vi "NF87xx.evt call STOP.vi"(0 "i ref in":refnum<vi>, 1 "Instance":string="N/A", 2 "System (N/A)":string="N/A", 5 "error in (no error)":errorcluster) -> (14 "i ref out":refnum<vi>, 19 "error out":errorcluster)   [LabVIEW 2014, in "NF87XX.lvlib"]
doc: "This VI sets the \"Stop\" case by a simple call. If \"System (N/A)\" is not connected (or \"N/A\" chosen), it acts on all systems connected to the instance, otherwise on the system only."
uses:
  NF87XX.lvlib
  CSCore/CSSystem/CoreLib/CoreLib.string 2 byte array.vi
  CSCore/BaseProcess/BaseProcess.lvlib
  CSCore/CSSystem/CoreLib/CoreLib.lvlib
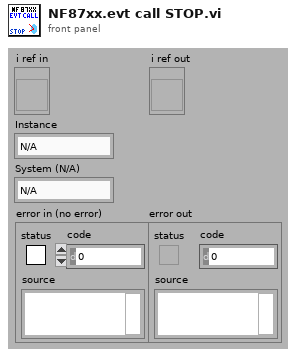
[diagram p1: front panel]
types:
  T1 = enum16{"simple", "synchronous", "asynchronous", "notification"}
  T2 = typedef "CoreDefs.rawDataType.ctl" = i8[]
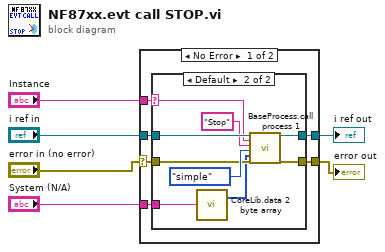
[diagram p0: block diagram]
diagram:
  n1 = case shown="No Error" "error in (no error)" {
    selector: "error in (no error)" -> [w8 w24]
    tunnel: [w12 w25] -> w6
    tunnel: [w11 w24] -> w5
    tunnel: "i ref in" -> [w10 w25]
    tunnel: "Instance" -> [w9 _]
    tunnel: "System (N/A)" -> [w7 _]
    frame No Error {
      n2 = case shown="Default" w9 {
        selector: w9 -> [_ w20]
        tunnel: [w14 w23] -> w12
        tunnel: [w13 w22] -> w11
        tunnel: w10 -> [w14 w21]
        tunnel: w8 -> [w13 w16]
        tunnel: w7 -> [_ w17]
        frame "N/A" {
        }
        frame Default {
          n3 = call-poly "CoreLib.data 2 byte array.vi"("string"=w17) -> ("byteArray out"=w15:T2)  [unwired: 18 in]
          n4 = call "BaseProcess.call process 1.vi"("i ref in"=w21, "Object"=w20, "Selector"="Stop", "CallType"=T1."simple", "Data"=w15, "error in (no error)"=w16) -> ("i ref out"=w23:refnum<vi>, "error out"=w22:errorcluster)  [unwired: 11 in, 1 out]
        }
      }
    }
    frame Error {
    }
  }
  "error out" <- w5
  "i ref out" <- w6
